vi "mapBlockGenerator.vi"(1 "Button Size":T1, 2 "Position":T2, 3 "Array":dbl[][](array[numeric])) -> (0 "output array":dbl[][](array[numeric]))   [LabVIEW 2014]
uses:
  <vilib>/Utility/miscctls.llb/LVPositionTypeDef.ctl
  <vilib>/Utility/miscctls.llb/LVBoundsTypeDef.ctl
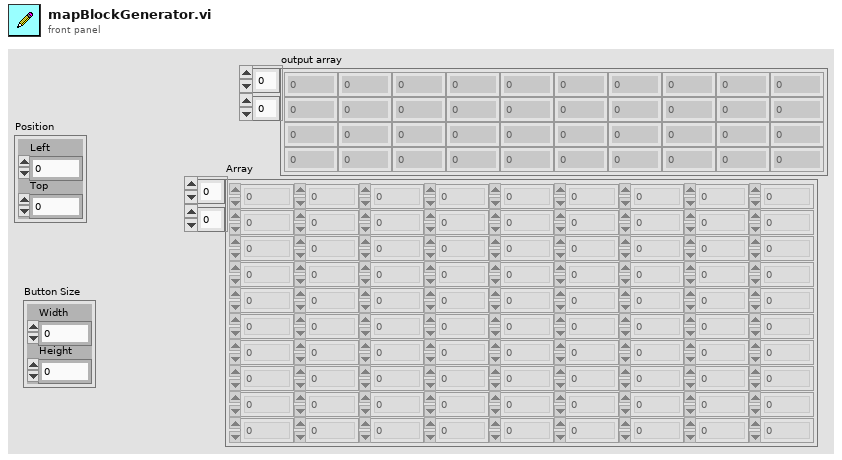
[diagram p1: front panel]
types:
  T1 = typedef "LVBoundsTypeDef.ctl" = cluster{"Width":u32, "Height":u32}
  T2 = typedef "LVPositionTypeDef.ctl" = cluster{"Left":i32, "Top":i32}
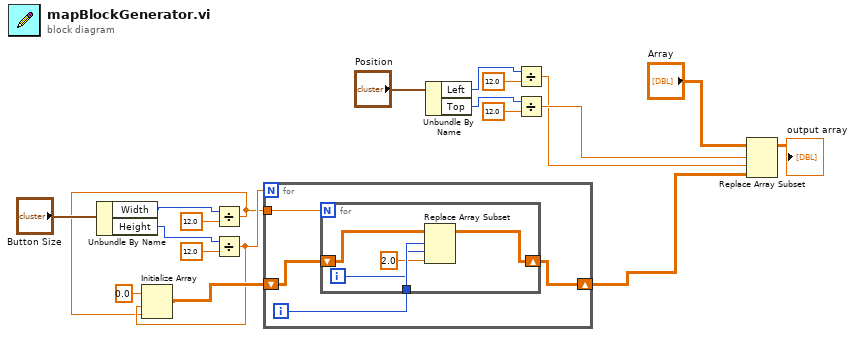
[diagram p0: block diagram]
diagram:
  n1 = Unbundle By Name("Button Size") -> ("Width"=w8:u32, "Height"=w7:u32)
  n2 = Divide(x=w8, y=12.0) -> (x/y=w2:dbl)
  n3 = Divide(x=w7, y=12.0) -> (x/y=w3:dbl)
  n4 = Initialize Array(0.0 ("element"), w3, w2) -> (w5:dbl[][])
  n5 = for {
    N: w3 -> [_]
    shift-right: [w22] -> w1
    shift-left: w5 -> [w23]
    tunnel: w2 -> [w20]
    i -> [w21]
    n6 = for {
      N: w20 -> [_]
      shift-right: [w27] -> w22
      shift-left: w23 -> [w28]
      tunnel: w21 -> [w26]
      i -> [w25]
      n7 = Replace Array Subset(array=w28, new element=2.0 ("new element/subarray"), index (row)=w26, index (col)=w25) -> (w27:dbl[][])
    }
  }
  n8 = Unbundle By Name("Position") -> ("Left"=w15:i32, "Top"=w14:i32)
  n9 = Divide(x=w15, y=12.0) -> (x/y=w12:dbl)
  n10 = Divide(x=w14, y=12.0) -> (x/y=w13:dbl)
  n11 = Replace Array Subset(array="Array", new element=w1, index (row)=w13, index (col)=w12) -> (→"output array":dbl[][])
